vi "Write U8 Array External.vi"(7 "Channel Index":i32, 8 "error in (no error)":errorcluster, 9 "Timeout (ms)":i32, 10 "U8 With Header":u8[](array[numeric]) format="%.0x", 11 "CIFCorePlugin in":refnum<class "CIFCorePlugin.lvclass">) -> (0 "error out":errorcluster, 1 "timed out?":bool, 3 "CIFCorePlugin out":refnum<class "CIFCorePlugin.lvclass">)   [LabVIEW 2021, in "CIFCorePlugin.lvclass"]
doc: "Write the full payload bytes, including the encoded header. This is intended for advanced applications where the full buffer was received externally. The header will still be updated with the new T_TX"
uses:
  CIFCorePlugin.lvclass
  CIFCorePlugin.lvclass/CIFCorePlugin.ctl
  <vilib>/CIF Foundation/CIF Channels Core/CIFChannels/CIFChannels.lvclass
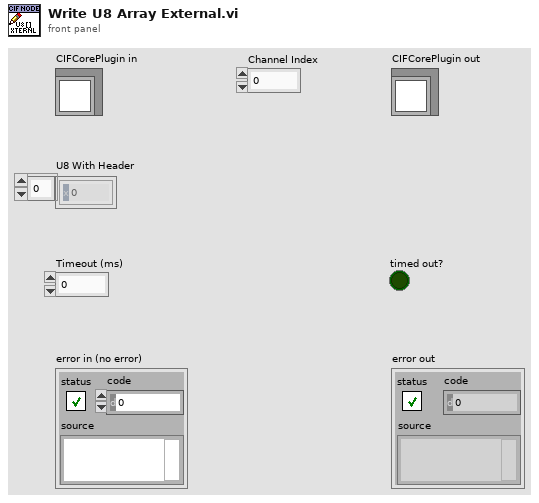
[diagram p1: front panel]
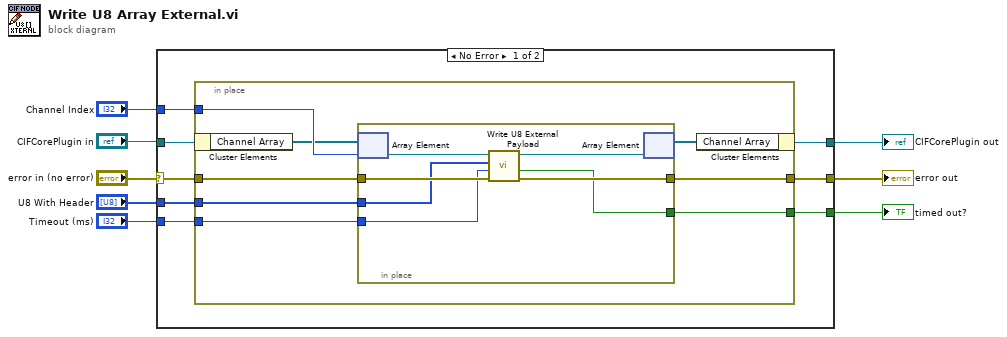
[diagram p0: block diagram]
diagram:
  n1 = case shown="No Error" "error in (no error)" {
    selector: "error in (no error)" -> [w16 w33]
    tunnel: [w15 w33] -> w6
    tunnel: [w13 w32] -> w7
    tunnel: "CIFCorePlugin in" -> [w14 w32]
    tunnel: "Channel Index" -> [w12 _]
    tunnel: "U8 With Header" -> [w11 _]
    tunnel: "Timeout (ms)" -> [w10 _]
    tunnel: [w9 _] -> w2
    frame No Error {
      n2 = in-place {
        in-place-border: w16 -> [w19]
        in-place-border: [w18] -> w15
        in-place-border: w12 -> [w24]
        in-place-border: w11 -> [w23]
        in-place-border: w10 -> [w22]
        in-place-border: [w21] -> w9
        n3 = in-place-cluster #1(w14) -> ("Channel Array"=w20:refnum<class "CIFChannels.lvclass">[])
        n4 = in-place {
          in-place-border: w19 -> [w30]
          in-place-border: [w29] -> w18
          in-place-border: w23 -> [w27]
          in-place-border: w22 -> [w26]
          in-place-border: [w25] -> w21
          n5 = in-place-array #2(w20, w24) -> (w31:refnum<class "CIFChannels.lvclass">)
          n6 = call-dynamic "Write U8 External Payload.vi"("error in (no error)"=w30, "Timeout (ms)"=w26, "U8 With Header in"=w27, "CIFChannels in"=w31) -> ("error out"=w29:errorcluster, "timed out?"=w25:bool, "CIFChannels out"=w28:refnum<class "CIFChannels.lvclass">)  [unwired: 4 in, 1 out]
          n7 = in-place-array #2(w28) -> (w17:refnum<class "CIFChannels.lvclass">[])  [unwired: 1 out]
        }
        n8 = in-place-cluster #1("Channel Array"=w17) -> (w13:refnum<class "CIFCorePlugin.lvclass">)
      }
    }
    frame Error {
    }
  }
  "error out" <- w6
  "CIFCorePlugin out" <- w7
  "timed out?" <- w2
